vi "Callback Change Data Type.vi"(6 "Variant":variant, 8 "error in (no error)":errorcluster, 9 "Old Values":string[][](array[string]), 10 "object ref in":T2, 11 "Table Change":T3) -> (0 "error out":errorcluster)   [LabVIEW 2013, in "tag bus configurable plugin editor node.lvclass"]
doc: "This VI gets called automatically when changes are made to the 'Data Type' column of the table and must handle changes appropriately. Register this callback using the appropriate 'Define Column' VI from the Table API."
uses:
  tag bus configurable plugin editor node.lvclass
  <vilib>/NI/DCAF/Tag Editor Core/Table API/Table Manager/Cell Change.ctl
  <vilib>/NI/DCAF/Tag Editor Core/Table API/Table Manager/object ref.ctl
  <vilib>/NI/DCAF/Tag Editor Core/Configuration Editor/Classes/Engine Parent/Engine Parent Editor Node.lvclass
  <vilib>/NI/DCAF/Tag Editor Core/Configuration Editor/Classes/Module editor node/module editor node.lvclass
  <vilib>/NI/Tag Bus/tag/Data Type.ctl
  module/configuration/tag bus configurable plugin module configuration.lvclass
  module/configuration/tag bus configurable plugin module configuration.lvclass/tag bus configurable plugin module configuration.ctl
  <vilib>/NI/Tag Bus/tag/tag descriptor.lvclass/tag descriptor.ctl
  <vilib>/NI/DCAF/Tag Editor Core/Table API/Table Manager.lvlib
  <vilib>/NI/Tag Bus/tag/tag descriptor.lvclass
  <vilib>/NI/DCAF/Tag Editor Core/Table API/Table Manager/Table Manager.lvclass
panel:
  in  "data type":T1
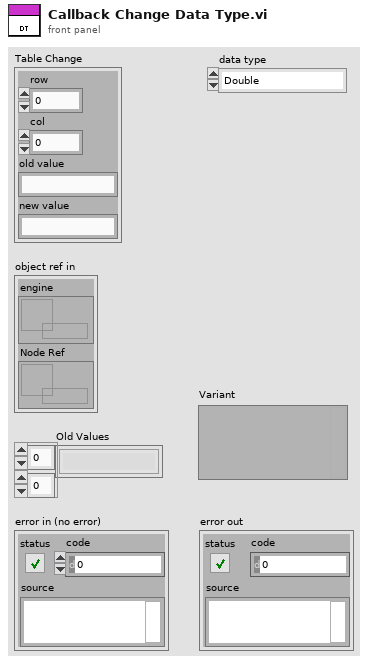
[diagram p1: front panel]
types:
  T1 = typedef "tag bus.lvlib/tag descriptor.lvclass/Data Type.ctl" = enum16{"Double", "Single", "I64", "I32", "I16", "I8", "U64", "U32", "U16", "U8", "Boolean", "String", "Array of Double", "Array of Single", "Array of I64", "Array of I32", "Array of I16", "Array of I8", "Array of U64", "Array of U32", "Array of U16", "Array of U8", "Array of Boolean", "Array of String"}
  T2 = typedef "Table Manager.lvlib/Table Manager.lvclass/object ref.ctl" = cluster{"engine":refnum<data-value>, "Node Ref":refnum<data-value>}
  T3 = typedef "Table Manager.lvlib/Cell Change.ctl" = cluster{"row":i32, "col":i32, "old value":string, "new value":string}
  T4 = typedef "tag bus configurable plugin module configuration.lvclass/Line.ctl" = cluster{"channel":refnum<class "TBM channel.lvclass">}
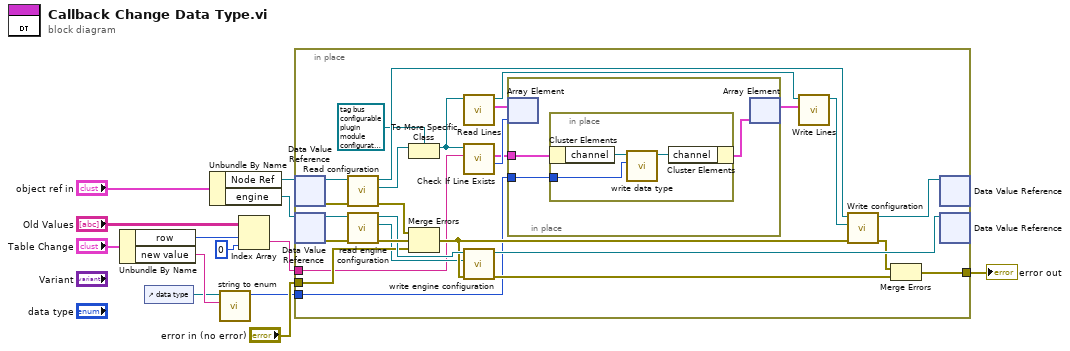
[diagram p0: block diagram]
diagram:
  n1 = Unbundle By Name("Table Change") -> ("row"=w5:i32, "new value"=w3:string)
  n2 = control-ref of="data type"() -> (w2:refnum<vi>)
  n3 = Unbundle By Name("object ref in") -> ("Node Ref"=w10:refnum<data-value>, "engine"=w9:refnum<data-value>)
  n4 = call <vilib>:"string to enum.vi"("String"=w3, "Enum"=w2) -> ("Value"=w1:i32)  [unwired: 8 in, 1 out]
  n5 = Index Array(array="Old Values", index (row)=w5, index (col)=0 ("disabled index (col)")) -> (element=w4:string)
  n6 = in-place {
    in-place-border: [w32] -> w13
    in-place-border: "error in (no error)" -> [w25]
    in-place-border: w4 -> [w16]
    in-place-border: w1 -> [w14]
    n7 = in-place-dvr #1(w10) -> (w29:refnum<class "module editor node.lvclass">, w31:errorcluster)
    n8 = in-place-dvr #2(w9) -> (w39:refnum<class "Engine Parent Editor Node.lvclass">, w40:errorcluster)
    n9 = call-dynamic "Read configuration.vi"("error in"=w31, "NISE_CEF_serializable node in"=w29) -> ("error out"=w30:errorcluster, "configuration"=w27:refnum<class "NISE_CEF_serializable configuration.lvclass">, "NISE_CEF_serializable node out"=w28:refnum<class "module editor node.lvclass">)  [unwired: 7 in]
    n10 = call <vilib>:"read engine configuration.vi"("error in"=w40, "Engine Parent Editor Node in"=w39) -> ("error out"=w36:errorcluster, "engine configuration"=w24:refnum<class "engine configuration.lvclass">, "Engine Parent Editor Node out"=w35:refnum<class "Engine Parent Editor Node.lvclass">)  [unwired: 7 in]
    n11 = To More Specific Class(target class=refnum<class "tag bus configurable plugin module configuration.lvclass"> refnum ("tag bus configurable plugin module configuration"), reference=w27) -> (specific class reference=w20:refnum<class "tag bus configurable plugin module configuration.lvclass">)  [unwired: 1 in, 1 out]
    n12 = Merge Errors(w30, w36, w25) -> (w26:errorcluster)
    n13 = call "Read Lines.vi"("tag bus configurable plugin module configuration in"=w20) -> ("Lines"=w19:T4[], "tag bus configurable plugin module configuration out"=w21:refnum<class "tag bus configurable plugin module configuration.lvclass">)  [unwired: 8 in, 1 out]
    n14 = call-dynamic "Check If Line Exists.vi"("Name to Locate"=w16, "tag bus configurable plugin module configuration in"=w20) -> ("Index"=w17:i32, "Line out"=w15:T4)  [unwired: 5 in, 3 out]
    n15 = call <vilib>:"write engine configuration.vi"("error in"=w26, "engine configuration"=w24, "Engine Parent Editor Node in"=w35) -> ("error out"=w34:errorcluster, "Engine Parent Editor Node out"=w38:refnum<class "Engine Parent Editor Node.lvclass">)  [unwired: 7 in]
    n16 = in-place {
      in-place-border: w15 -> [w43]
      in-place-border: w14 -> [w42]
      n17 = in-place-array #3(w19, w17) -> ()  [unwired: 1 out]
      n18 = in-place {
        in-place-border: w42 -> [w44]
        n19 = in-place-cluster #4(w43) -> ("channel"=w46:refnum<class "TBM channel.lvclass">)
        n20 = call <vilib>:"write data type.vi"("data type"=w44, "system tag in"=w46) -> ("system tag out"=w45:refnum<class "TBM channel.lvclass">)  [unwired: 8 in, 1 out]
        n21 = in-place-cluster #4("channel"=w45) -> (w41:T4)
      }
      n22 = in-place-array #3(w41) -> (w18:T4[])  [unwired: 1 out]
    }
    n23 = call "Write Lines.vi"("Lines"=w18, "tag bus configurable plugin module configuration in"=w21) -> ("tag bus configurable plugin module configuration out"=w22:refnum<class "tag bus configurable plugin module configuration.lvclass">)  [unwired: 8 in, 1 out]
    n24 = call-dynamic "Write configuration.vi"("error in"=w26, "configuration"=w22, "NISE_CEF_serializable node in"=w28) -> ("error out"=w33:errorcluster, "NISE_CEF_serializable node out"=w37:refnum<class "module editor node.lvclass">)  [unwired: 7 in]
    n25 = Merge Errors(w33, w34) -> (w32:errorcluster)
    n26 = in-place-dvr #1(w37) -> ()  [unwired: 2 out]
    n27 = in-place-dvr #2(w38) -> ()  [unwired: 2 out]
  }
  "error out" <- w13
